vi "自动索引.vi"() -> ()   [LabVIEW 2010]
panel:
  out "波形图表":i32(graph)
  out "累积数组":i32[][](array[numeric])
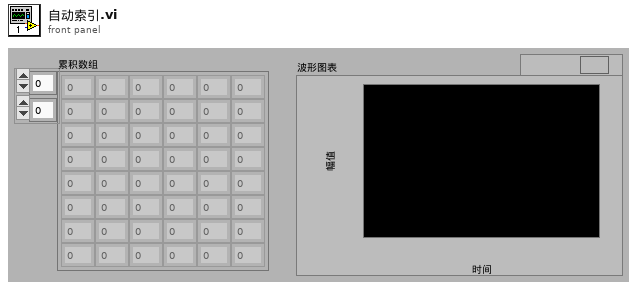
[diagram p1: front panel]
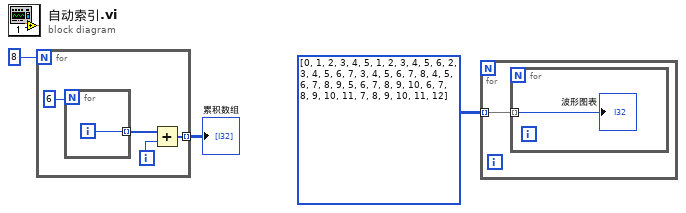
[diagram p0: block diagram]
diagram:
  n1 = for {
    N: 8 -> [_]
    tunnel: [w5] -> w1 mode=indexing
    i -> [w4]
    n2 = for {
      N: 6 -> [_]
      tunnel: [w8] -> w6 mode=indexing
      i -> [w8]
    }
    n3 = Add(x=w6, y=w4) -> (x+y=w5:i32[])
  }
  "累积数组" <- w1
  n4 = for {
    tunnel: i32[][] [[0, 1, 2, 3, 4, 5], [1, 2, 3, 4, 5, 6], [2, 3, 4, 5, 6, 7], [3, 4, 5, 6, 7, 8], [4, 5, 6, 7, 8, 9], [5, 6, 7, 8, 9, 10], [6, 7, 8, 9, 10, 11], [7, 8, 9, 10, 11, 12]] ("累加数组") -> [w9] mode=indexing
    n5 = for {
      tunnel: w9 -> [w10] mode=indexing
      "波形图表" <- w10
    }
  }
